vi "PXI-Wait for Stale AI Data Bank.vi"(8 "error in (no error)":errorcluster, 10 "timeout (ms)":i32=5000) -> (0 "error out":errorcluster={"status"=TRUE, "code"=555, "source"="Timed out waiting for Signal Bank."})   [LabVIEW 2020]
uses:
  PXI Globals.vi
panel:
  out "Numeric":i32
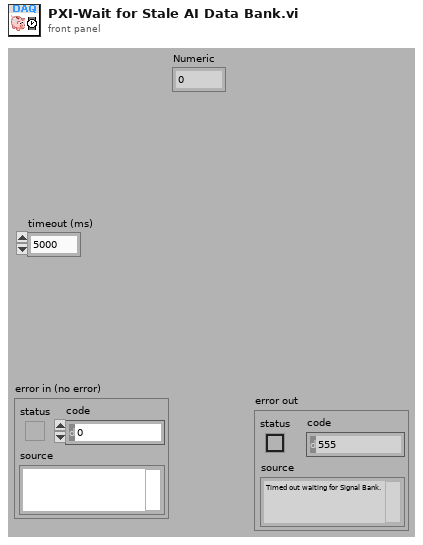
[diagram p1: front panel]
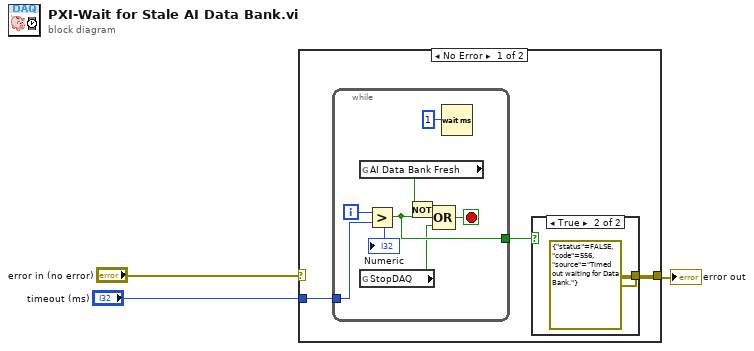
[diagram p0: block diagram]
diagram:
  n1 = case shown="No Error" "error in (no error)" {
    selector: "error in (no error)" -> [_ w16]
    tunnel: [w5 w16] -> w3
    tunnel: "timeout (ms)" -> [w4 _]
    frame No Error {
      n2 = while {
        tunnel: w4 -> [w10]
        tunnel: [w11] -> w6
        i -> [w12]
        stop <- w14 stop-if-true
        n3 = global read "PXI Globals.vi" "AI Data Bank Fresh"() -> (w13:bool)
        n4 = global read "PXI Globals.vi" "StopDAQ"() -> (w9:bool)
        n5 = Greater?(x=w12, y=w10) -> (0:w11:bool)
        n6 = Not(x=w13) -> (.not. x?=w8:bool)
        n7 = Compound Arithmetic op=OR(w8, w11, w9) -> (w14:bool)
        n8 = Wait (ms)(milliseconds to wait=1) -> ()  [unwired: 1 out]
        "Numeric" <- w12
      }
      n9 = case shown="True" w6 {
        tunnel: [_ errorcluster {"status"=FALSE, "code"=556, "source"="Timed out waiting for Data Bank."} ("error out 2")] -> w5
        frame False {
        }
        frame True {
        }
      }
    }
    frame Error {
    }
  }
  "error out" <- w3
